vi "Ctor.vi"(8 "error in (no error)":errorcluster) -> (0 "error out":errorcluster, 3 "GVIWebProcessorApp out":refnum<class "GVIWebProcessorApp.lvclass">)   [LabVIEW 2020, in "PicoG-Processor.lvlib" / "GVIWebProcessorApp.lvclass"]
uses:
  GVIWebProcessorApp.lvclass
  Ref Data.ctl
  UI Refs.ctl
  <vilib>/Utility/miscctls.llb/LVRectTypeDef.ctl
  GVIWebProcessorApp.lvclass/GVIWebProcessorApp.ctl
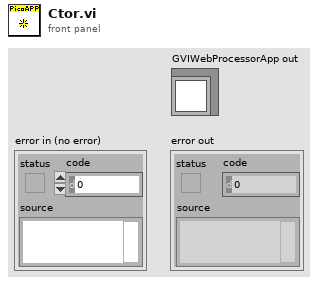
[diagram p1: front panel]
types:
  T1 = typedef "PicoG-Processor.lvlib/GVIWebProcessorApp.lvclass/Ref Data.ctl" = cluster{"hWnd":i32, "UI Refs":T2, "Collapsed":bool, "Async Anim Ref":refnum<vi>, "Expanded Bounds":T3, "Expanding":bool, "Collapsing":bool}
  T2 = typedef "PicoG-Processor.lvlib/GVIWebProcessorApp.lvclass/UI Refs.ctl" = cluster{"Main Window":refnum<vi>, "List Panel":refnum<vi>, "H Splitter":refnum<vi>, "V Splitter":refnum<vi>, "Open Project":refnum<vi>, "Project Name":refnum<vi>}
  T3 = typedef "LVRectTypeDef.ctl" = cluster{"Left":i16, "Top":i16, "Right":i16, "Bottom":i16}
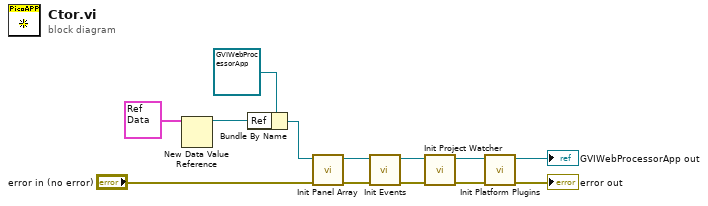
[diagram p0: block diagram]
diagram:
  n1 = New Data Value Reference(data value=T1 {"hWnd"=0, "UI Refs"={"Main Window"=refnum, "List Panel"=refnum, "H Splitter"=refnum, "V Splitter"=refnum, "Open Project"=refnum, "Project Name"=refnum}, "Collapsed"=FALSE, "Async Anim Ref"=refnum, "Expanded Bounds"={"Left"=0, "Top"=0, "Right"=0, "Bottom"=0}, "Expanding"=FALSE, "Collapsing"=FALSE} ("Ref Data")) -> (data value reference=w11:refnum<data-value>)  [unwired: 1 in, 1 out]
  n2 = Bundle By Name(cluster=refnum<class "GVIWebProcessorApp.lvclass"> refnum ("GVIWebProcessorApp in"), "Ref"=w11) -> (w9:refnum<class "GVIWebProcessorApp.lvclass">)
  n3 = call "Init Panel Array.vi"("error in (no error)"="error in (no error)", "GVIWebProcessorApp in"=w9) -> ("error out"=w7:errorcluster, "GVIWebProcessorApp out"=w8:refnum<class "GVIWebProcessorApp.lvclass">)  [unwired: 8 in]
  n4 = call "Init Events.vi"("error in (no error)"=w7, "GVIWebProcessorApp in"=w8) -> ("error out"=w5:errorcluster, "GVIWebProcessorApp out"=w6:refnum<class "GVIWebProcessorApp.lvclass">)  [unwired: 8 in]
  n5 = call "Init Project Watcher.vi"("error in (no error)"=w5, "GVIWebProcessorApp in"=w6) -> ("error out"=w3:errorcluster, "GVIWebProcessorApp out"=w4:refnum<class "GVIWebProcessorApp.lvclass">)  [unwired: 8 in]
  n6 = call "Init Platform Plugins.vi"("error in (no error)"=w3, "GVIWebProcessorApp in"=w4) -> ("error out"=→"error out":errorcluster, "GVIWebProcessorApp out"=→"GVIWebProcessorApp out":refnum<class "GVIWebProcessorApp.lvclass">)  [unwired: 8 in]
